vi "SRV_VERSION.vi"() -> (0 "SRV Version":string)   [LabVIEW 2009]
doc: "Contains the version of the software to display on GUIs.\n\n\nAuthor: Mike Schultz - Logic PD"
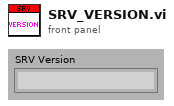
[diagram p1: front panel]
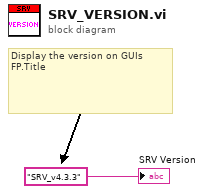
[diagram p0: block diagram]
diagram:
  # "Display the version on GUIs\nFP.Title"
  "SRV Version" <- "SRV_v4.3.3" ("Front Panel Window:Title")
